vi "(SubVI) Calculate Center-Mean QPD from oneside or twoside data_YCC.vi"(0 "Stage Array (um)":dbl[](array[numeric]), 1 "QPD Array (V)":dbl[](array[numeric]), 2 "Center Stage (um)":dbl, 3 "avg range for QPD center (nm)":dbl=600.0) -> (6 "Center QPD (V)":dbl format="%0.2f")   [LabVIEW 2014]
uses:
  <vilib>/Analysis/baseanly.llb/Mean (DBL).vi
  <vilib>/Analysis/NI_AALBase.lvlib
panel:
  out "Center index":dbl
  out "Right bound index":dbl
  out "Left bound index":dbl
  out "To right? (+)":bool
  out "To left? (-)":bool
  # "20181117\nYCC"
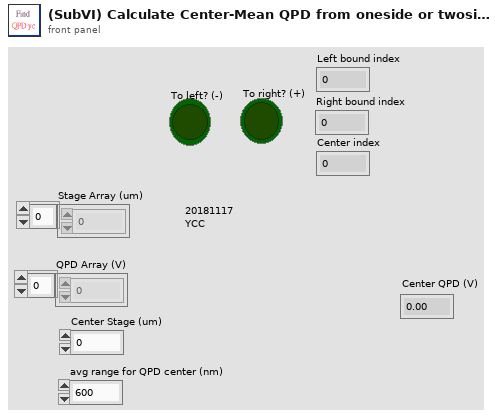
[diagram p1: front panel]
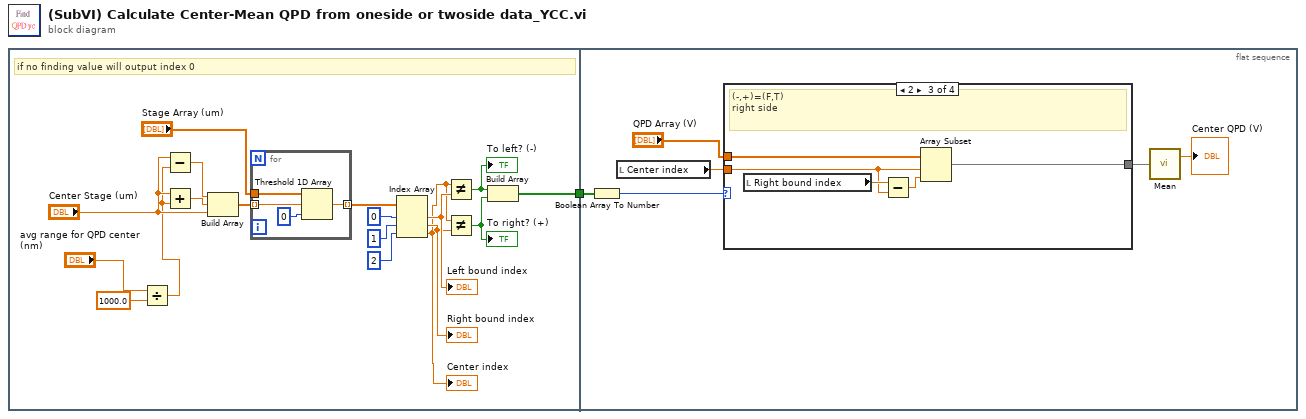
[diagram p0: block diagram]
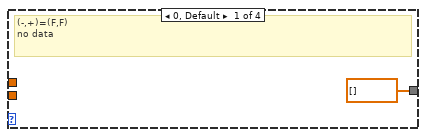
[diagram p2: hidden frame]
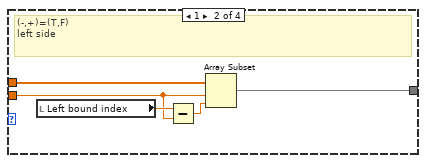
[diagram p3: hidden frame]
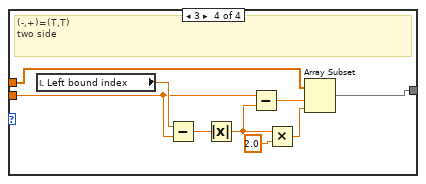
[diagram p4: hidden frame]
diagram:
  n1 = flat-sequence {
    tunnel: [w9] -> w1
    tunnel: w1 -> [w29]
    frame #0 {
      # "if no finding value will output index 0"
      n2 = Divide(x="avg range for QPD center (nm)", y=1000.0) -> (x/y=w3:dbl)
      n3 = Subtract(x="Center Stage (um)", y=w3) -> (x-y=w18:dbl)
      n4 = Add(x="Center Stage (um)", y=w3) -> (x+y=w17:dbl)
      n5 = Build Array(w18, w17, "Center Stage (um)") -> (w16:dbl[])
      n6 = for {
        tunnel: [w23] -> w15 mode=indexing
        tunnel: "Stage Array (um)" -> [w22]
        tunnel: w16 -> [w21] mode=indexing
        n7 = Threshold 1D Array(1:0 ("start index (0)"), 2:w21, 3:w22) -> (0:w23:dbl)
      }
      n8 = Index Array(array=w15, index #1=0 ("index"), index #2=1 ("index"), index #3=2 ("index")) -> (element #1=w12:dbl, element #2=w8:dbl, element #3=w2:dbl)
      "Left bound index" <- w12
      "Right bound index" <- w8
      "Center index" <- w2
      n9 = Not Equal?(x=w2, y=w12) -> (x != y?=w11:bool)
      "To left? (-)" <- w11
      n10 = Not Equal?(x=w2, y=w8) -> (x != y?=w10:bool)
      "To right? (+)" <- w10
      n11 = Build Array(w11, w10) -> (w9:bool[])
    }
    frame #1 {
      n12 = Boolean Array To Number(Boolean array=w29) -> (number=w28:u32)
      n13 = local read "Center index"() -> (w26:dbl)
      n14 = case shown="2" w28 {
        tunnel: "QPD Array (V)" -> [_ w35 w40 w49]
        tunnel: w26 -> [_ w33 w37 w46]
        tunnel: [dbl[] [] w31 w36 w41] -> w25
        frame 0, Default {
          # "(-,+)=(F,F)\nno data"
        }
        frame 1 {
          # "(-,+)=(T,F)\nleft side"
          n15 = local read "Left bound index"() -> (w34:dbl)
          n16 = Subtract(x=w34, y=w33) -> (x-y=w32:dbl)
          n17 = Array Subset(array=w35, index=w33, length=w32) -> (w31:dbl[])
        }
        frame 2 {
          # "(-,+)=(F,T)\nright side"
          n18 = local read "Right bound index"() -> (w39:dbl)
          n19 = Subtract(x=w39, y=w37) -> (x-y=w38:dbl)
          n20 = Array Subset(array=w40, index=w37, length=w38) -> (w36:dbl[])
        }
        frame 3 {
          # "(-,+)=(T,T)\ntwo side"
          n21 = local read "Left bound index"() -> (w48:dbl)
          n22 = Subtract(x=w48, y=w46) -> (x-y=w47:dbl)
          n23 = Absolute Value(x=w47) -> (abs(x)=w44:dbl)
          n24 = Subtract(x=w46, y=w44) -> (x-y=w45:dbl)
          n25 = Multiply(x=w44, y=2.0) -> (x*y=w42:dbl)
          n26 = Array Subset(array=w49, index=w45, length=w42) -> (w41:dbl[])
        }
      }
      n27 = call-poly <vilib>:"Mean.vi"("X"=w25) -> ("mean"=→"Center QPD (V)":dbl)  [unwired: 1 out]
    }
  }
